vi "FT_Get_Queue_Status.vi"(0 "Handle":u32) -> (1 "FT_Status":u32, 2 "Bytes Waiting":u32)   [LabVIEW 2017]
uses:
  FTD2XX.dll
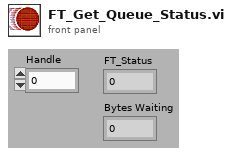
[diagram p1: front panel]
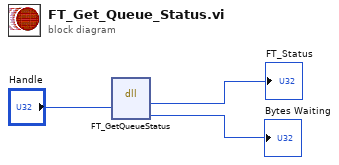
[diagram p0: block diagram]
diagram:
  n1 = dll-call lib="FTD2XX.dll" fn="FT_GetQueueStatus"("Handle"="Handle") -> ("FT_Status"=→"FT_Status":u32, "BytesWaiting"=→"Bytes Waiting":u32)  [unwired: 5 in, 2 out]
